vi "Same.vi"() -> (0 "error out":errorcluster)   [LabVIEW 2017, in "Assertions.Tests.lvlib" / "Assert Equal.lvlib"]
uses:
  Assert Equal.lvlib
  src/Transparent Assertions/Constraints/IsEqual/Create.vi
  src/Transparent Assertions/Constraints/IsEqual/IsEqual.lvclass
  src/Transparent Assertions/Assertions/Assertions.lvlib
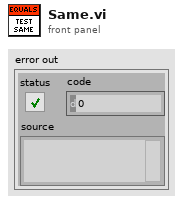
[diagram p1: front panel]
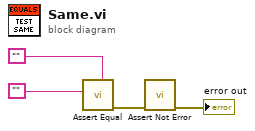
[diagram p0: block diagram]
diagram:
  n1 = call "Assert Equal.vi"("Expected"="", "Actual"="") -> ("error out"=w2:errorcluster)  [unwired: 9 in]
  n2 = call "Assert Not Error.vi"("error in (no error)"=w2) -> ("error out"=→"error out":errorcluster)  [unwired: 10 in]
